vi "Log State.vi"(8 "error in":errorcluster, 10 "Model Status":T3, 11 "Data":T1) -> (0 "error out":errorcluster, 3 "Data out":T1)   [LabVIEW 2015, in "Logger.lvlib"]
uses:
  Logger.lvlib
  Model/TypeDefs/Get Model Status Control.ctl
  TypeDefs/Logger Data.ctl
  TypeDefs/Logger State.ctl
  Model/Model.lvlib
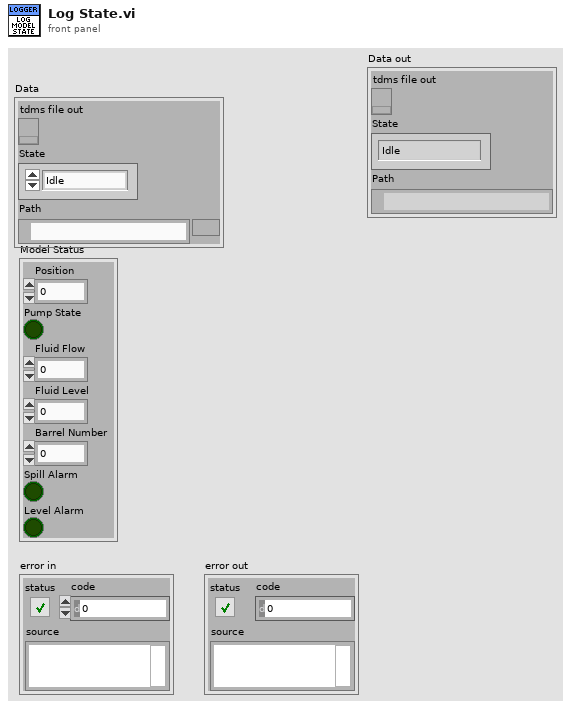
[diagram p1: front panel]
types:
  T1 = typedef "Logger.lvlib/Logger Data.ctl" = cluster{"tdms file out":refnum<k34>, "State":T2, "Path":path}
  T2 = typedef "Logger.lvlib/Logger State.ctl" = enum16{"Idle", "Working"}
  T3 = typedef "Model.lvlib/Get Model Status Control.ctl" = cluster{"Position":dbl, "Pump State":bool, "Fluid Flow":dbl, "Fluid Level":dbl, "Barrel Number":i32, "Spill Alarm":bool, "Level Alarm":bool}
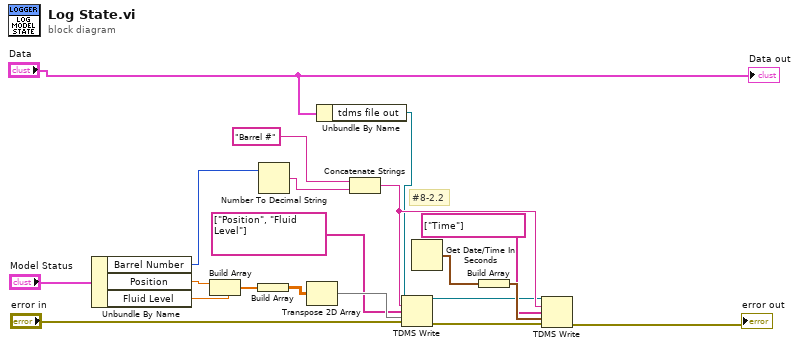
[diagram p0: block diagram]
diagram:
  # "#8-2.2"
  n1 = Unbundle By Name("Model Status") -> ("Barrel Number"=w15:i32, "Position"=w7:dbl, "Fluid Level"=w6:dbl)
  n2 = Build Array(w7, w6) -> (w5:dbl[])
  n3 = Build Array(w5) -> (w2:dbl[][])
  n4 = Number To Decimal String(number=w15) -> (decimal integer string=w14:string)  [unwired: 1 in]
  n5 = Transpose 2D Array(2D array=w2) -> (transposed array=w4:dbl[][])
  n6 = Unbundle By Name("Data") -> ("tdms file out"=w11:refnum<k34>)
  n7 = Concatenate Strings("Barrel #" ("string"), w14) -> (w12:string)
  n8 = TDMS Write(0:w11, 5:w12, 7:string[] ["Position", "Fluid Level"] ("channel name(s) in (Untitled)"), 9:w4, 11:"error in") -> (4:w1:refnum<k34>, 15:w18:errorcluster)  [unwired: 1 in, 2 out]
  n9 = Get Date/Time In Seconds() -> (seconds since 1Jan1904=w10:timestamp)
  n10 = Build Array(w10) -> (w9:timestamp[])
  n11 = TDMS Write(0:w1, 5:w12, 7:string[] ["Time"] ("channel name(s) in (Untitled)"), 9:w9, 11:w18) -> (15:→"error out":errorcluster)  [unwired: 1 in, 3 out]
  "Data out" <- "Data"
